vi "Untitled 1.vi"() -> ()   [LabVIEW 2023]
panel:
  out "Signal[V]":dbl(knob) scale=0.0..10.0
  out "High":bool
  out "Low":bool
  out "Pumpa":bool
  in  "Signal [mA]":dbl(knob) scale=4.0..20.0
  out "Nivo[m]":dbl(slide) scale=0.0..5.0
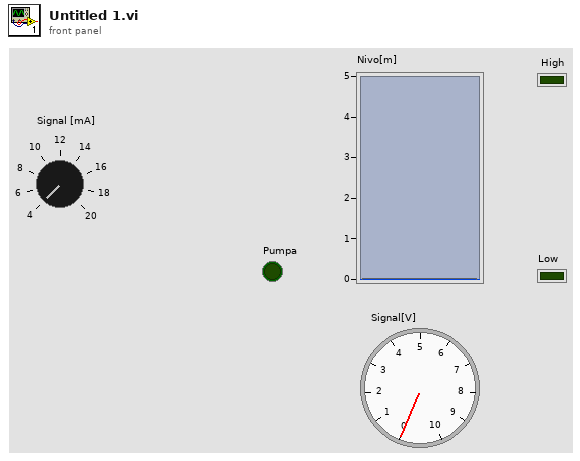
[diagram p1: front panel]
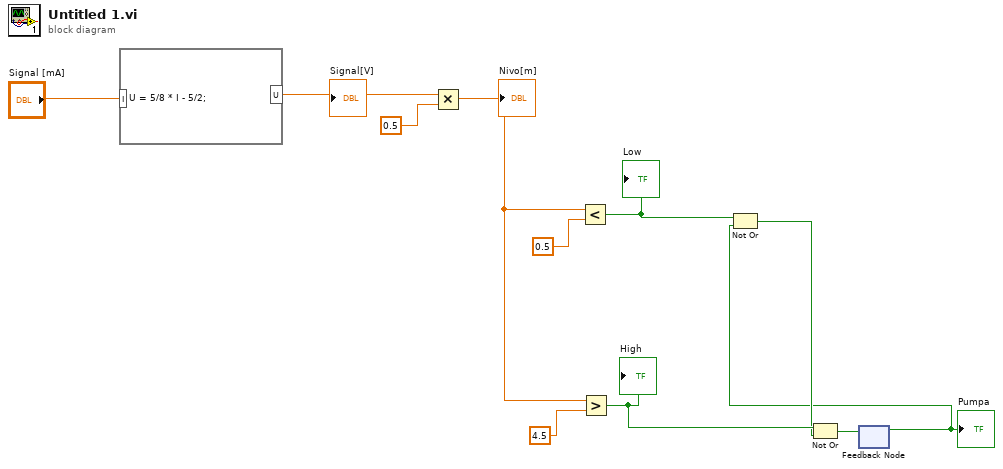
[diagram p0: block diagram]
diagram:
  n1 = formula code="U = 5/8 * I - 5/2;"("I"="Signal [mA]") -> ("U"=w10:dbl)
  "Signal[V]" <- w10
  n2 = Multiply(x=w10, y=0.5) -> (x*y=w7:dbl)
  "Nivo[m]" <- w7
  n3 = Less?(x=w7, y=0.5) -> (x < y?=w4:bool)
  "Low" <- w4
  n4 = Greater?(x=w7, y=4.5) -> (0:w5:bool)
  "High" <- w5
  n5 = feedback #1() -> (w1:bool)  [unwired: 1 in]
  "Pumpa" <- w1
  n6 = Not Or(1:w1, 2:w4) -> (0:w3:bool)
  n7 = Not Or(1:w3, 2:w5) -> (0:w2:bool)
  n8 = feedback-in #1(w2) -> ()
